vi "ustalRuchPoziomy.vi"(6 "Wybór komory":T3, 9 "Czy na żądanej pozycji?":bool, 10 "Ruch wstepny":T1, 11 "Faza ruchu":T2) -> (2 "Stan poziomy":T1, 3 "Faza ruchu poziomego":T2)   [LabVIEW 2014]
uses:
  parametryKomorVIs/WyborKomory.ctl
  RuchPoziomy.ctl
  Faza_ruchu.ctl
  AkcjaGFV.ctl
  timerRuchuPoziomegoVIs/Czynnosc.ctl
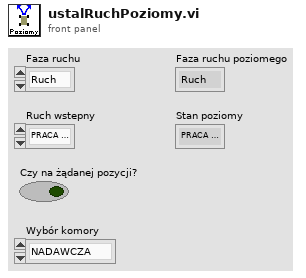
[diagram p1: front panel]
types:
  T1 = typedef "RuchPoziomy.ctl" = enum16{"PRACA RĘCZNA", "LEWO", "PRAWO", "WYŁ."}
  T2 = typedef "Faza_ruchu.ctl" = enum16{"Ruch", "Poczekaj", "Pomiar"}
  T3 = typedef "WyborKomory.ctl" = enum16{"NADAWCZA", "ODBIORCZA"}
  T4 = typedef "WejsciaParametry.ctl" = cluster{"LEWO":bool, "PRAWO":bool, "GORA":bool, "DOL":bool, "Praca reczna":bool, "Stop":bool, "Start":bool, "Komora":bool, "Wyjscie":bool, "Rodzaj pomiarow":T5, "Czas pomiaru [s]":dbl, "Czas inicjalizacji ramion [s]":dbl, "Liczba punktów":i32, "Liczba płaszczyzn":i32}
  T5 = typedef "RodzajPomiarow.ctl" = enum16{"Izolacyjność Akustyczna ISO 10140", "Losowanie punktów", "Sekwencja testowa"}
  T6 = typedef "Czynnosc.ctl" = enum16{"reset all", "działaj"}
  T7 = typedef "AkcjaGFV.ctl" = enum16{"Czytaj", "Zapisz", "Reset"}
  T8 = typedef "Gotowosc.ctl" = cluster{"Poziomy":bool, "Pionowy":bool}
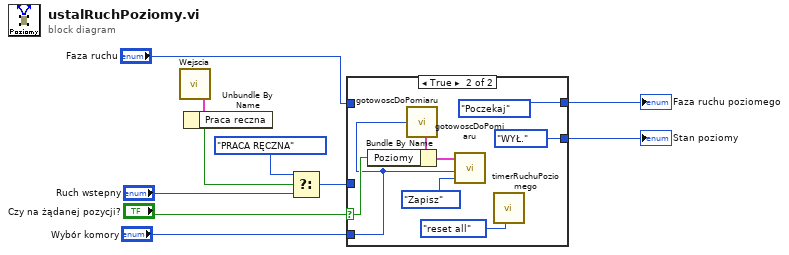
[diagram p0: block diagram]
diagram:
  n1 = call "Wejscia.vi"() -> ("Wyjście"=w8:T4)  [unwired: 5 in]
  n2 = Unbundle By Name(w8) -> ("Praca reczna"=w6:bool)
  n3 = Select(t=RuchPoziomy."PRACA RĘCZNA" ("Stan pracy ręcznej - poz"), s=w6, f="Ruch wstepny") -> (s? t:f=w1:T1)
  n4 = case shown="True" "Czy na żądanej pozycji?" {
    selector: "Czy na żądanej pozycji?" -> [_ w17]
    tunnel: "Faza ruchu" -> [w12 _]
    tunnel: [w12 Faza_ruchu."Poczekaj" ("f")] -> w4
    tunnel: w1 -> [w11 _]
    tunnel: [w11 RuchPoziomy."WYŁ." ("Stan poziomy")] -> w2
    tunnel: "Wybór komory" -> [_ w14]
    frame False {
    }
    frame True {
      n5 = call "gotowoscDoPomiaru.vi"("Wybór komory"=w14) -> ("Gotowość wyjście"=w15:T8)  [unwired: 4 in]
      n6 = Bundle By Name(cluster=w15, "Poziomy"=w17) -> (w19:T8)
      n7 = call "gotowoscDoPomiaru.vi"("Akcja"=AkcjaGFV."Zapisz", "Wybór komory"=w14, "Gotowość"=w19) -> ()  [unwired: 2 in, 1 out]
      n8 = call "timerRuchuPoziomego.vi"("Czynność"=Czynnosc."reset all") -> ()  [unwired: 10 in, 1 out]
    }
  }
  "Faza ruchu poziomego" <- w4
  "Stan poziomy" <- w2
